vi "1-read-fichierSRC.vi"(4 "err in":errorcluster) -> (0 "err out":errorcluster, 2 "fichier src":path, 3 "tdms file out":refnum<k34>)   [LabVIEW 2010, in "lv_04.lvlib"]
uses:
  lv_04.lvlib
  SRC_var_globale.vi
panel:
  out "Chemin TDMS":path=path "D:/_fo_sys/ni_prj/applis/src_2.tdms"
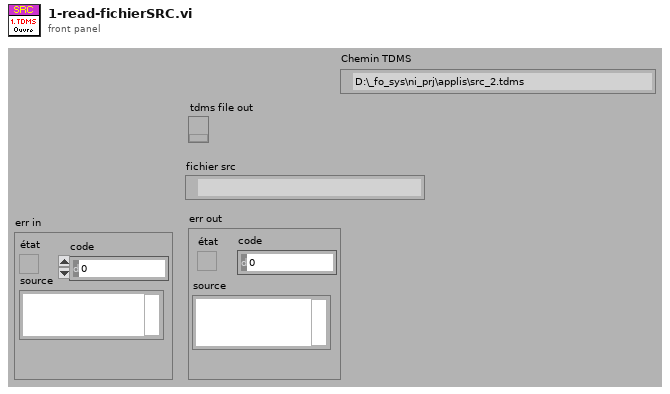
[diagram p1: front panel]
types:
  T1 = enum16{"open", "open or create", "create or replace", "create", "open (read-only)"}
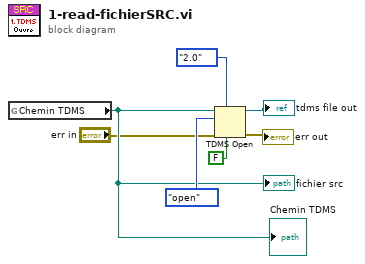
[diagram p0: block diagram]
diagram:
  n1 = global read "SRC_var_globale.vi" "Chemin TDMS"() -> (w2:path)
  "fichier src" <- w2
  "Chemin TDMS" <- w2
  n2 = TDMS Open(6:FALSE ("disable buffering (T)"), 7:enum16{"1.0", "2.0"}."2.0" ("file format version (2.0)"), 8:"err in", 10:T1."open" ("operation"), 11:w2) -> (0:→"err out":errorcluster, 3:→"tdms file out":refnum<k34>)  [unwired: 1 in]
